vi "Calculate Average Stage Current.vi"(8 "error in (no error)":errorcluster, 11 "Stage Waveform Section":dbl[](array[numeric])) -> (0 "error out":errorcluster, 3 "Average Stage Current out":dbl)   [LabVIEW 2015, in "Fuel Injection Addon Engine.lvlib"]
uses:
  Fuel Injection Addon Engine.lvlib
  <vilib>/Analysis/baseanly.llb/Mean (DBL).vi
  <vilib>/Analysis/NI_AALBase.lvlib
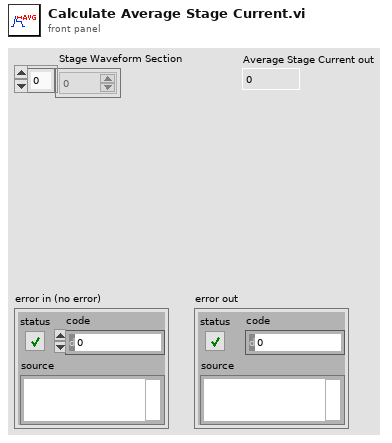
[diagram p1: front panel]
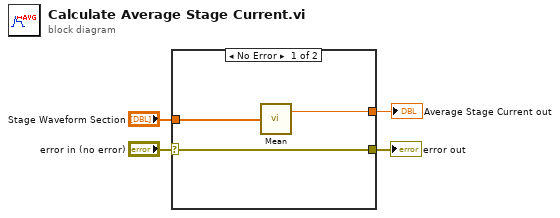
[diagram p0: block diagram]
diagram:
  n1 = case shown="No Error" "error in (no error)" {
    selector: "error in (no error)" -> [w6 w8]
    tunnel: "Stage Waveform Section" -> [w7 _]
    tunnel: [w6 w8] -> w2
    tunnel: [w5 _] -> w1
    frame No Error {
      n2 = call-poly <vilib>:"Mean.vi"("X"=w7) -> ("mean"=w5:dbl)  [unwired: 1 out]
    }
    frame Error {
    }
  }
  "error out" <- w2
  "Average Stage Current out" <- w1
